vi "test.vi"() -> ()   [LabVIEW 2014]
uses:
  Zhensheng/documents/GitHub/zsLV/ctl/pose.ctl
  <vilib>/Tufts CEEO ROS for LabVIEW Software/ROS/Code/Console/Servers/ServerSubs/TopicDef.ctl
  <vilib>/Tufts CEEO ROS for LabVIEW Software/ROS/Code/SubVIs/_ROSDirection.ctl
  Zhensheng/documents/GitHub/zsLV/ctl/Point.ctl
  Zhensheng/documents/GitHub/zsLV/ctl/RPY.ctl
panel:
  in  "停止":bool
  out "输出簇":T1
  out "msg out":string
  out "Quaternion":cluster{"x":dbl, "y":dbl, "z":dbl, "w":dbl}
  out "error out":errorcluster
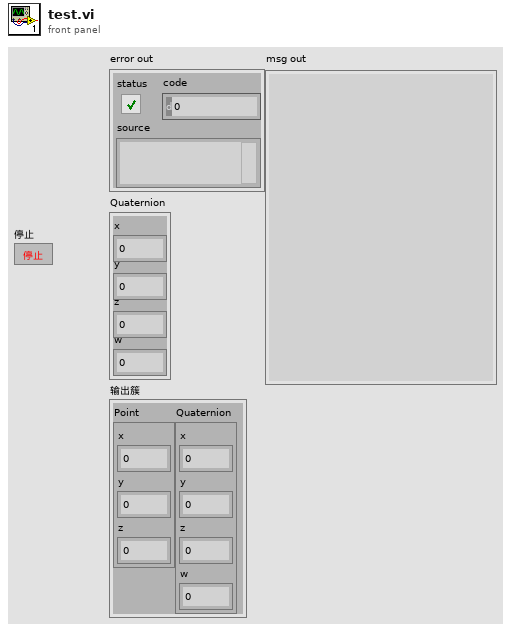
[diagram p1: front panel]
types:
  T1 = typedef "pose.ctl" = cluster{"Point":cluster{"x":dbl, "y":dbl, "z":dbl}, "Quaternion":cluster{"x":dbl, "y":dbl, "z":dbl, "w":dbl}}
  T2 = typedef "TopicDef.ctl" = cluster{"Topic":string, "Type":string, "Action":T3, "Update (ms)":u16, "queue size":u16}
  T3 = typedef "_ROSDirection.ctl" = enum16{"Node", "Publisher", "Subscriber", "ServiceClient", "ServiceProvider"}
  T4 = typedef "_ROSControl.ctl" = cluster{"topic port":u16, "Node":string, "topic":string, "type":string, "node port":u16, "error ":errorcluster, "Direction":T3, "Update (ms)":u16, "FIFO size":u16}
  T5 = typedef "RPY.ctl" = cluster{"Roll (y)":dbl, "Pitch (x)":dbl, "Yaw (z)":dbl}
  T6 = typedef "Point.ctl" = cluster{"x":dbl, "y":dbl, "z":dbl}
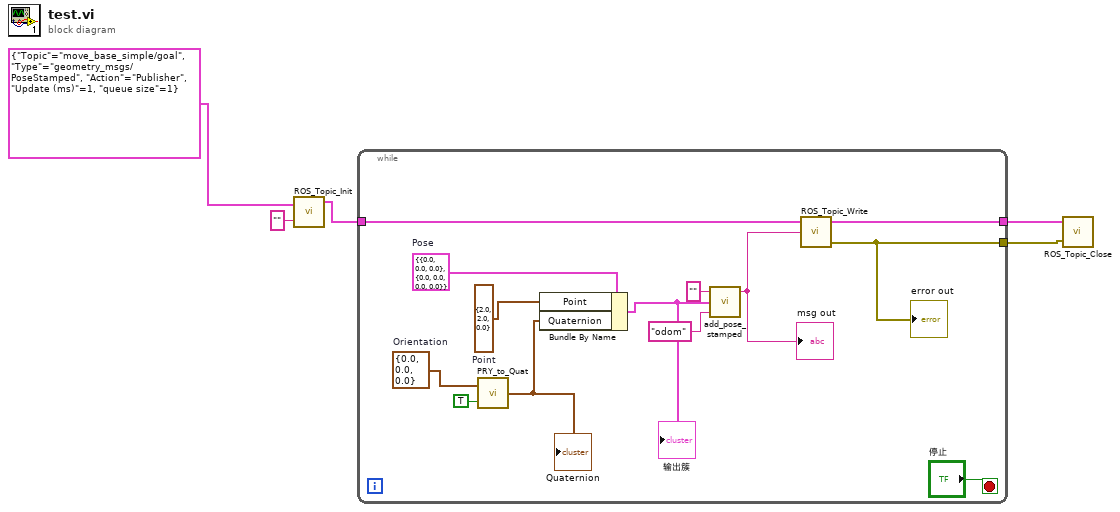
[diagram p0: block diagram]
diagram:
  n1 = call <vilib>:"ROS_Topic_Init.vi"("Definitions"=T2 {"Topic"="move_base_simple/goal", "Type"="geometry_msgs/PoseStamped", "Action"=enum."Publisher", "Update (ms)"=1, "queue size"=1}, "node"="") -> ("ROS out"=w1:T4)  [unwired: 1 in, 1 out]
  n2 = while {
    tunnel: [w18] -> w5
    tunnel: [w17] -> w4
    tunnel: w1 -> [w7]
    stop <- "停止" stop-if-true
    w15 = T5 {"Roll (y)"=0.0, "Pitch (x)"=0.0, "Yaw (z)"=0.0}  # Orientation
    w13 = T6 {"x"=2.0, "y"=2.0, "z"=0.0}  # Point
    w14 = T1 {"Point"={"x"=0.0, "y"=0.0, "z"=0.0}, "Quaternion"={"x"=0.0, "y"=0.0, "z"=0.0, "w"=0.0}}  # Pose
    n3 = call <vilib>:"PRY_to_Quat.vi"("From Degrees? (T)"=TRUE, "Orientation"=w15) -> ("Quaternion"=w12:cluster{"x":dbl, "y":dbl, "z":dbl, "w":dbl})
    "Quaternion" <- w12
    n4 = Bundle By Name(cluster=w14, "Point"=w13, "Quaternion"=w12) -> (w11:T1)
    "输出簇" <- w11
    n5 = call <vilib>:"add_pose_stamped.vi"("frame_id"="odom", "Pose"=w11, "msg in"="") -> ("msg out"=w9:string)  [unwired: 2 in]
    "msg out" <- w9
    n6 = call <vilib>:"ROS_Topic_Write.vi"("Msg in"=w9, "ROS in"=w7) -> ("error out"=w18:errorcluster, "ROS out"=w17:T4)  [unwired: 2 in]
    "error out" <- w18
  }
  n7 = call <vilib>:"ROS_Topic_Close.vi"("error in"=w5, "ROS in"=w4) -> ()  [unwired: 2 in, 1 out]
